vi "DS BaseActor PollingTime.vi"() -> ()   [LabVIEW 2015, in "CS++Utilities.lvlib"]
doc: "Activate or deactivate CS++PVProxy when using DataSocket."
uses:
  CS++Utilities.lvlib
panel:
  out "Polling Mode":i32=-1
  in  "PollingMode URL":string="dstp://localhost/CSPP_Core_SV/myBaseActor_PollingMode"
  in  "Stop Button":bool
  in  "PollingTime URL":string="dstp://localhost/CSPP_Core_SV/myBaseActor_PollingTime"
  out "Polling Interval":dbl[unit]
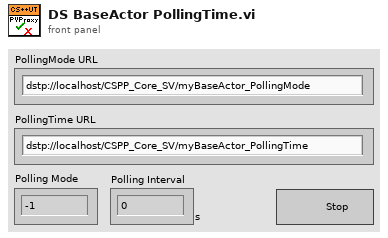
[diagram p1: front panel]
types:
  T1 = enum16{"Read", "Write", "ReadWrite", "BufferedRead", "BufferedReadWrite"}
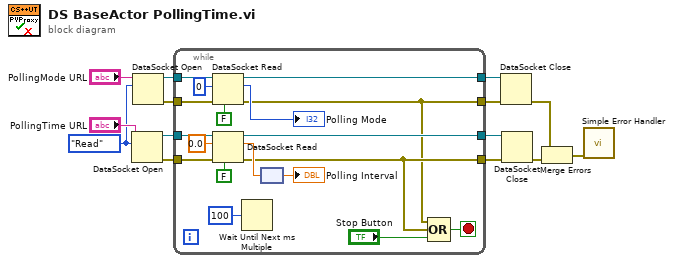
[diagram p0: block diagram]
diagram:
  w7 = T1."Read" ("mode")
  n1 = DataSocket Open(10:w7, 11:"PollingTime URL") -> (0:w13:errorcluster, 3:w12:refnum<k13>)  [unwired: 2 in]
  n2 = DataSocket Open(10:w7, 11:"PollingMode URL") -> (0:w5:errorcluster, 3:w6:refnum<k13>)  [unwired: 2 in]
  n3 = while {
    tunnel: w6 -> [w21]
    tunnel: w5 -> [w20]
    tunnel: [w17] -> w4
    tunnel: [w16] -> w3
    tunnel: w13 -> [w32]
    tunnel: [w24] -> w11
    tunnel: w12 -> [w31]
    tunnel: [w30] -> w10
    stop <- w25 stop-if-true
    n4 = DataSocket Read(6:FALSE ("wait for updated value (T)"), 8:w20, 10:0, 11:w21) -> (0:w16:errorcluster, 2:→"Polling Mode":i32, 3:w17:refnum<k13>)  [unwired: 1 in, 4 out]
    n5 = DataSocket Read(6:FALSE ("wait for updated value (T)"), 8:w32, 10:0.0 ("Polling Interval"), 11:w31) -> (0:w24:errorcluster, 2:w28:dbl, 3:w30:refnum<k13>)  [unwired: 1 in, 4 out]
    n6 = Wait Until Next ms Multiple(millisecond multiple=u32 100) -> ()  [unwired: 1 out]
    n7 = node(w28) -> (→"Polling Interval":dbl[unit])
    n8 = Compound Arithmetic op=OR(w16, w24, "Stop Button") -> (w25:bool)
  }
  n9 = DataSocket Close(8:w3, 11:w4) -> (0:w1:errorcluster)  [unwired: 1 in, 1 out]
  n10 = DataSocket Close(8:w11, 11:w10) -> (0:w9:errorcluster)  [unwired: 1 in, 1 out]
  n11 = Merge Errors(w1, w9) -> (w2:errorcluster)
  n12 = call <vilib>:"Simple Error Handler.vi"("error in (no error)"=w2) -> ()  [unwired: 4 in, 5 out]
